vi "AI Vibration Data.vi"(10 "Enum":enum16{"Read", "Write"}(ring), 11 "Vibration Data":waveform(dbl)[](array[waveform])) -> (3 "Vibration Data":waveform(dbl)[](array[waveform]))   [LabVIEW 2022 SP3]
panel:
  out "error out":errorcluster
  in  "error in":errorcluster
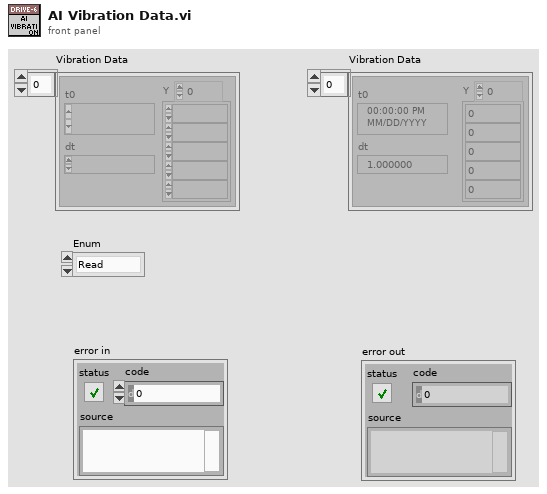
[diagram p1: front panel]
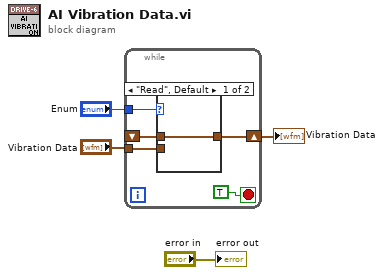
[diagram p0: block diagram]
diagram:
  n1 = while {
    tunnel: "Enum" -> [w9]
    tunnel: "Vibration Data" -> [w7]
    shift-right: [w6] -> w1
    shift-left: _ -> [w5]
    stop <- TRUE stop-if-true
    n2 = case shown="\"Read\", Default" w9 {
      tunnel: w7 -> [_ w11]
      tunnel: [w10 w11] -> w6
      tunnel: w5 -> [w10 _]
      frame "Read", Default {
      }
      frame "Write" {
      }
    }
  }
  "Vibration Data" <- w1
  "error out" <- "error in"
